vi "Stop Acquisition.vi"(8 "error in (no error)":errorcluster, 11 "Picam in":refnum<class "Picam.lvclass">) -> (0 "error out":errorcluster, 3 "Picam out":refnum<class "Picam.lvclass">)   [LabVIEW 2019, in "Picam.lvclass"]
uses:
  Picam.lvclass
  Picam.lvclass/Picam.ctl
  picam32_LabView_SDK/PICam_lib/PICam.lvlib
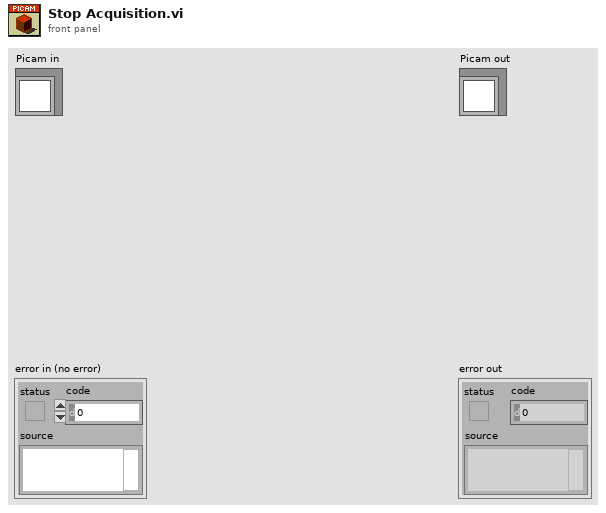
[diagram p1: front panel]
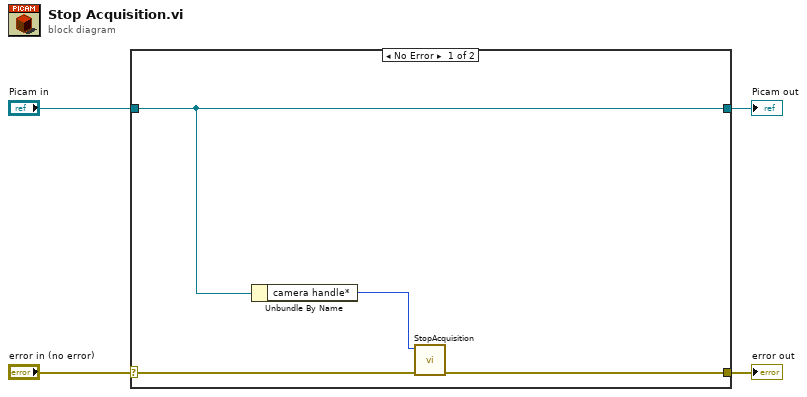
[diagram p0: block diagram]
diagram:
  n1 = case shown="No Error" "error in (no error)" {
    selector: "error in (no error)" -> [w8 w10]
    tunnel: [w7 w10] -> w3
    tunnel: [w6 w9] -> w1
    tunnel: "Picam in" -> [w6 w9]
    frame No Error {
      n2 = Unbundle By Name(w6) -> ("camera handle*"=w5:u64)
      n3 = call "StopAcquisition.vi"("error in"=w8, "camera handle in"=w5) -> ("error out"=w7:errorcluster)  [unwired: 8 in, 1 out]
    }
    frame Error {
    }
  }
  "error out" <- w3
  "Picam out" <- w1
